vi "Select Device.vi"(8 "error in (no error)":errorcluster, 11 "Device":i32) -> (0 "error out":errorcluster, 3 "function return":i32)   [LabVIEW 2020, in "ThorECU.lvlib"]
doc: "long SelectDevice(const long Device);"
uses:
  ThorECU.lvlib
  ThorECU.dll
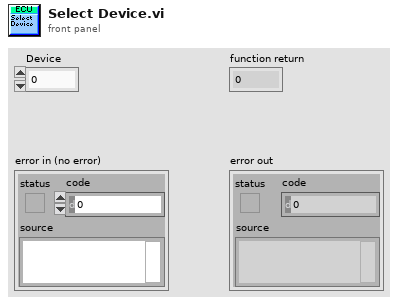
[diagram p1: front panel]
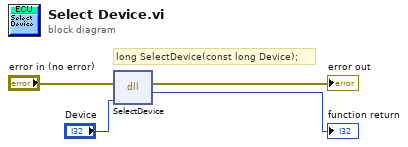
[diagram p0: block diagram]
diagram:
  # "long SelectDevice(const long Device);"
  n1 = dll-call lib="D:/software/TweezerTron Project/Instruments/Thorlabs/ECU_SDK/ThorECU.*" fn="SelectDevice"(error in="error in (no error)", "Device"="Device") -> (error out=→"error out":errorcluster, →"function return":i32)  [unwired: 3 in, 1 out]
